vi "FWHM_Sigma.vi"(8 "error in (no error)":errorcluster caption="entrée d'erreur (pas d'erreur)", 11 "Acq Cam Basler en entrée":refnum<class "Acq Cam Basler.lvclass">) -> (0 "error out":errorcluster caption="sortie d'erreur", 3 "Acq Cam Basler en sortie":refnum<class "Acq Cam Basler.lvclass">)   [LabVIEW 2023, in "Acq Cam Basler.lvclass"]
uses:
  Acq Cam Basler.lvclass
  Acq Cam Basler.lvclass/Acq Cam Basler.ctl
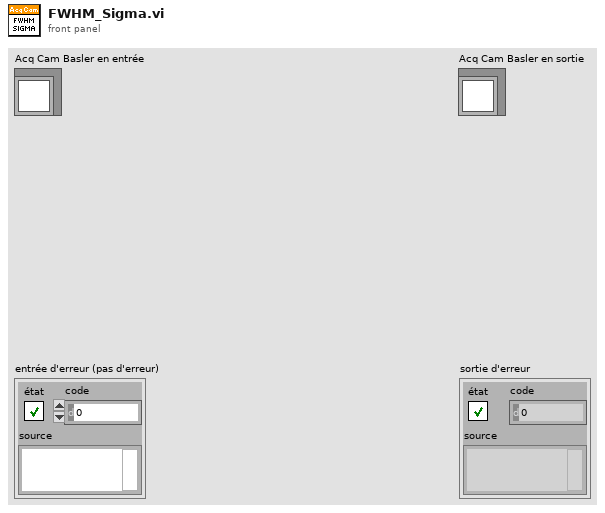
[diagram p1: front panel]
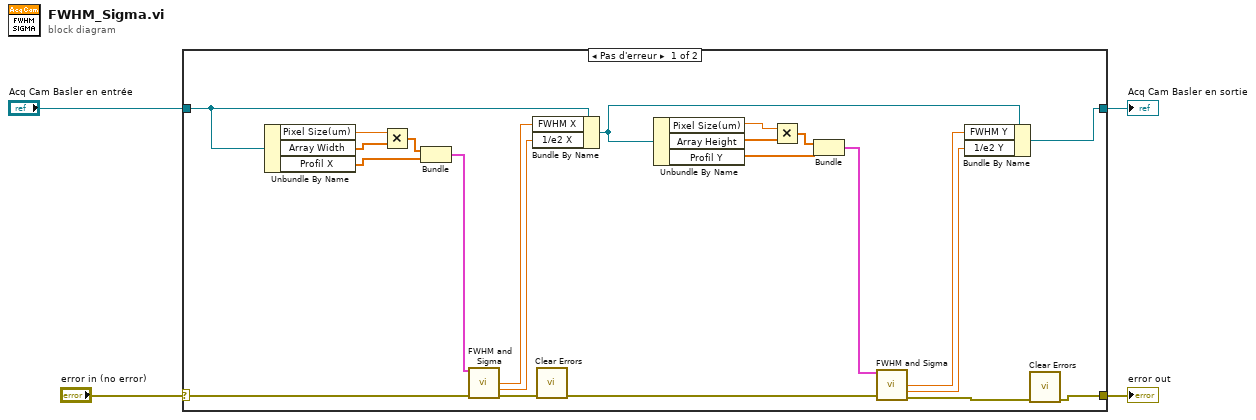
[diagram p0: block diagram]
diagram:
  n1 = case shown="Pas d'erreur" "error in (no error)" {
    selector: "error in (no error)" -> [w24 w28]
    tunnel: [w22 w28] -> w3
    tunnel: [w7 w27] -> w1
    tunnel: "Acq Cam Basler en entrée" -> [w16 w27]
    frame No Error {
      n2 = Unbundle By Name(w16) -> ("Pixel Size(um)"=w21:dbl, "Array Width"=w20:dbl[], "Profil X"=w18:dbl[])
      n3 = Multiply(x=w21, y=w20) -> (x*y=w19:dbl[])
      n4 = Bundle(w19, "Profil X"=w18) -> (w17:cluster{dbl[], "Profil X":dbl[]})  [unwired: 1 in]
      n5 = call <vilib>:"FWHM and Sigma.vi"("Data in"=w17, "error in"=w24) -> ("FWHM"=w10:dbl, "1/e^2 width"=w9:dbl, "error out"=w26:errorcluster)  [unwired: 9 in, 2 out]
      n6 = Bundle By Name(cluster=w16, "FWHM X"=w10, "1/e2 X"=w9) -> (w8:refnum<class "Acq Cam Basler.lvclass">)
      n7 = call <vilib>:"Clear Errors.vi"("error in (no error)"=w26) -> ("error out"=w23:errorcluster)  [unwired: 5 in, 1 out]
      n8 = Unbundle By Name(w8) -> ("Pixel Size(um)"=w15:dbl, "Array Height"=w14:dbl[], "Profil Y"=w12:dbl[])
      n9 = Multiply(x=w15, y=w14) -> (x*y=w13:dbl[])
      n10 = Bundle(w13, "Profil Y"=w12) -> (w11:cluster{dbl[], "Profil Y":dbl[]})  [unwired: 1 in]
      n11 = call <vilib>:"FWHM and Sigma.vi"("Data in"=w11, "error in"=w23) -> ("FWHM"=w6:dbl, "1/e^2 width"=w5:dbl, "error out"=w25:errorcluster)  [unwired: 9 in, 2 out]
      n12 = Bundle By Name(cluster=w8, "FWHM Y"=w6, "1/e2 Y"=w5) -> (w7:refnum<class "Acq Cam Basler.lvclass">)
      n13 = call <vilib>:"Clear Errors.vi"("error in (no error)"=w25) -> ("error out"=w22:errorcluster)  [unwired: 5 in, 1 out]
    }
    frame Error {
    }
  }
  "error out" <- w3
  "Acq Cam Basler en sortie" <- w1
